vi "Get EM Gain Range.vi"(10 "high":i32, 11 "low":i32) -> (1 "function return":u32, 2 "high out":i32, 3 "low out":i32)   [LabVIEW 2018, in "Copy of Andor SDK.lvlib"]
doc: "EXPNETTYPE unsigned int WINAPI GetEMGainRange(int * low, int * high);"
uses:
  Copy of Andor SDK.lvlib
  <userlib>/Andor SDK/ATMCD32D.dll
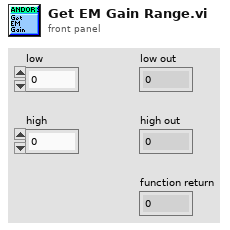
[diagram p1: front panel]
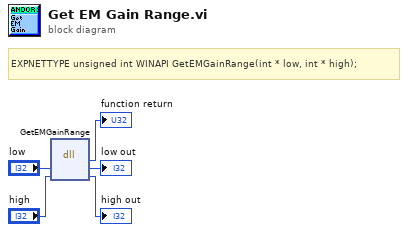
[diagram p0: block diagram]
diagram:
  # "EXPNETTYPE unsigned int WINAPI GetEMGainRange(int * low, int * high);"
  n1 = dll-call lib="C:/Program Files (x86)/National Instruments/LabVIEW 2018/user.lib/Andor SDK/ATMCD32D.*" fn="GetEMGainRange"("low"="low", "high"="high") -> (→"function return":u32, "low"=→"low out":i32, "high"=→"high out":i32)  [unwired: 3 in, 2 out]
